vi "Write Elevator Location.vi"(8 "error in (no error)":errorcluster, 10 "Elevator Position":string, 11 "Display Console in":refnum<class "Display Console.lvclass">) -> (0 "error out":errorcluster, 3 "Display Console out":refnum<class "Display Console.lvclass">)   [LabVIEW 2019, in "Display Console Actor.lvlib" / "Display Console.lvclass"]
uses:
  Display Console.lvclass
  Display Console.lvclass/Display Console.ctl
  Abstract Display Console Actor/Abstract Display Console Actor/Abstract Display Console.lvclass
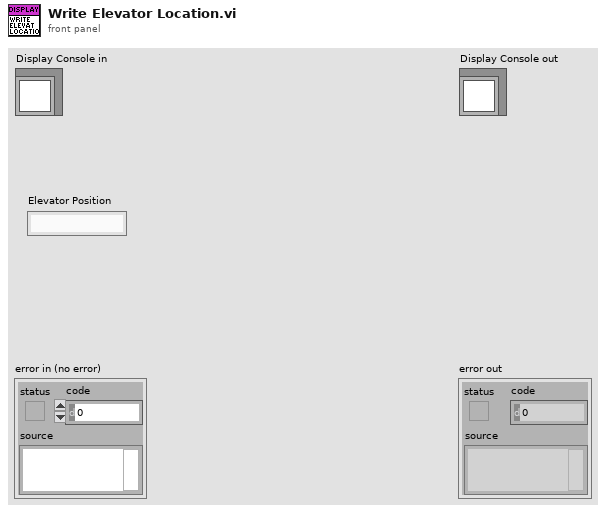
[diagram p1: front panel]
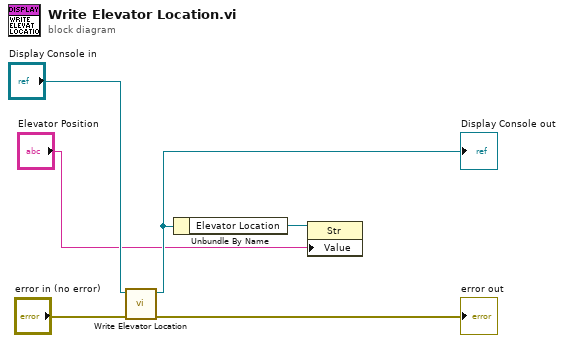
[diagram p0: block diagram]
diagram:
  n1 = call-parent "Write Elevator Location.vi"("error in (no error)"="error in (no error)", "Abstract Display Console in"="Display Console in") -> ("error out"=→"error out":errorcluster, "Abstract Display Console out"=w2:refnum<class "Display Console.lvclass">)  [unwired: 8 in]
  "Display Console out" <- w2
  n2 = Unbundle By Name(w2) -> ("Elevator Location"=w3:refnum<vi>)
  n3 = property class="Str"(reference=w3, "Value"="Elevator Position") -> ()  [unwired: 1 in, 2 out]
